vi "read_params.vi"(8 "error in (no error)":errorcluster, 11 "SpectralBiclustering in":refnum<class "SpectralBiclustering.lvclass">) -> (0 "error out":errorcluster, 2 "params":T1={"n_clusters"={"n_clusters_type"="int", "n_clusters_int"=3.0, "n_clusters_list"=[]}, "method"="bistochastic", "n_components"=6.0, "n_best"=3.0, "svd_method"="randomized", "n_svd_vecs"={"n_svd_vecs_type"="None", "n_svd_int"=0.0}, "mini_batch"=FALSE, "init"={"init_type"="k-means++", "init_list"=[]}, "random_state"=0.0}, 3 "SpectralBiclustering out":refnum<class "SpectralBiclustering.lvclass">)   [LabVIEW 2020, in "SpectralBiclustering.lvclass"]
uses:
  SpectralBiclustering.lvclass
  Controls/spectral_biclustering_params.ctl
  SpectralBiclustering.lvclass/SpectralBiclustering.ctl
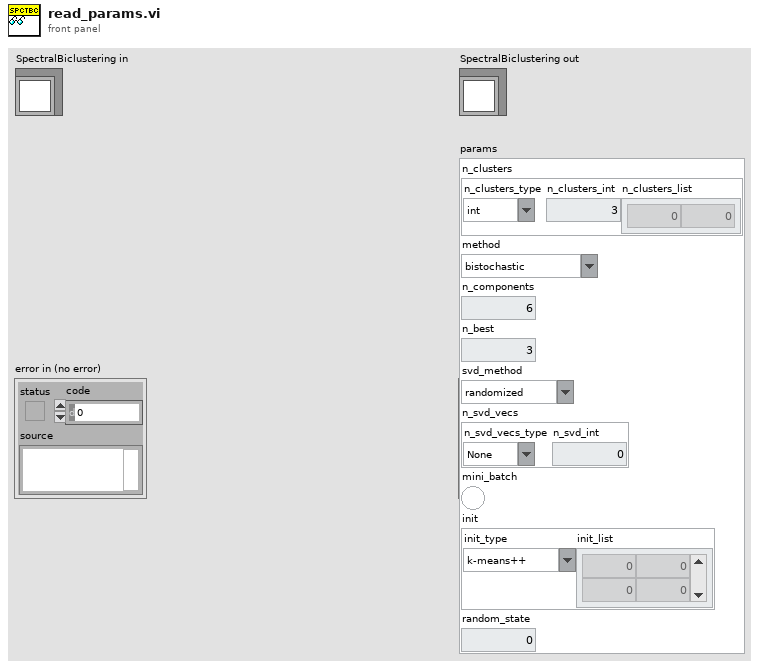
[diagram p1: front panel]
types:
  T1 = typedef "spectral_biclustering_params.ctl" = cluster{"n_clusters":cluster{"n_clusters_type":string, "n_clusters_int":dbl, "n_clusters_list":dbl[]}, "method":string, "n_components":dbl, "n_best":dbl, "svd_method":string, "n_svd_vecs":cluster{"n_svd_vecs_type":string, "n_svd_int":dbl}, "mini_batch":bool, "init":cluster{"init_type":string, "init_list":dbl[][]}, "random_state":dbl}
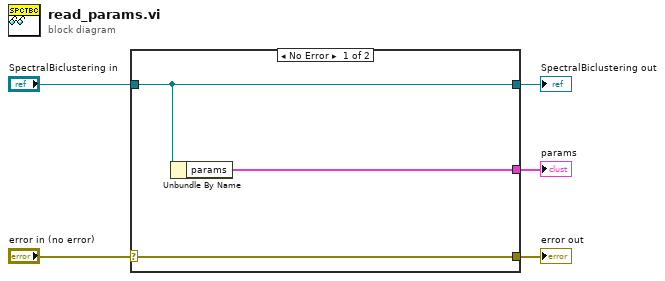
[diagram p0: block diagram]
diagram:
  n1 = case shown="No Error" "error in (no error)" {
    selector: "error in (no error)" -> [w8 w9]
    tunnel: [w8 w9] -> w4
    tunnel: [w7 w10] -> w2
    tunnel: "SpectralBiclustering in" -> [w7 w10]
    tunnel: [w6 _] -> w1
    frame No Error {
      n2 = Unbundle By Name(w7) -> ("params"=w6:T1)
    }
    frame Error {
    }
  }
  "error out" <- w4
  "SpectralBiclustering out" <- w2
  "params" <- w1
